vi "validate classes.vi"(6 "Child":refnum<class>, 8 "error in":errorcluster, 11 "Parent":refnum<class>) -> (0 "error out":errorcluster, 1 "class name":string, 3 "unique parent name":string)   [LabVIEW 2020, in "Publisher Subscriber.lvlib"]
uses:
  Publisher Subscriber.lvlib
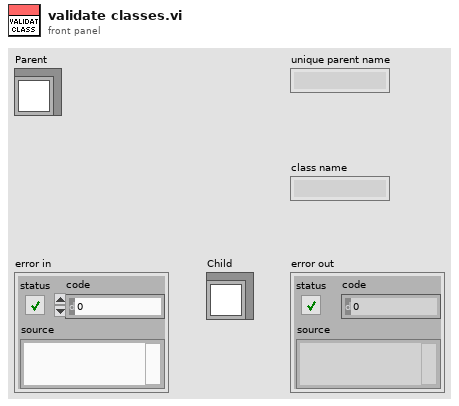
[diagram p1: front panel]
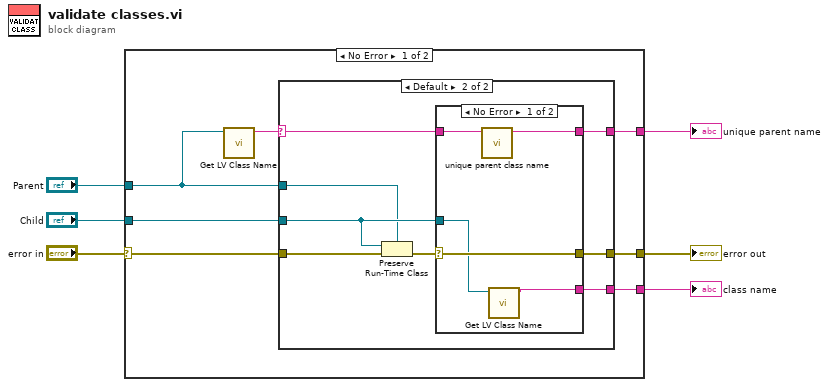
[diagram p0: block diagram]
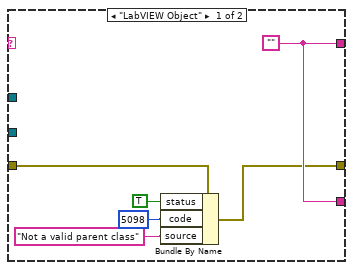
[diagram p2: hidden frame]
diagram:
  n1 = case shown="No Error" "error in" {
    selector: "error in" -> [w7 w34]
    tunnel: [w12 _] -> w6
    tunnel: "Child" -> [w11 _]
    tunnel: [w10 w34] -> w4
    tunnel: "Parent" -> [w9 _]
    tunnel: [w8 _] -> w2
    frame No Error {
      n2 = call <vilib>:"Get LV Class Name.vi"("object"=w9) -> ("class name"=w13:string)  [unwired: 9 in, 1 out]
      n3 = case shown="Default" w13 {
        selector: w13 -> [_ w27]
        tunnel: [w19 w24] -> w12
        tunnel: w11 -> [_ w23]
        tunnel: [w18 w22] -> w10
        tunnel: w9 -> [_ w20]
        tunnel: [w19 w26] -> w8
        tunnel: w7 -> [w17 w25]
        frame "LabVIEW Object" {
          w19 = ""
          n4 = Bundle By Name(cluster=w17, "status"=TRUE, "code"=5098, "source"="Not a valid parent class") -> (w18:errorcluster)
        }
        frame Default {
          n5 = Preserve Run-Time Class(object in=w23, error in=w25, 2:w20) -> (error out=w21:errorcluster)  [unwired: 1 out]
          n6 = case shown="No Error" w21 {
            selector: w21 -> [w29 w33]
            tunnel: w27 -> [w32 _]
            tunnel: [w31 _] -> w26
            tunnel: [w30 _] -> w24
            tunnel: w23 -> [w28 _]
            tunnel: [w29 w33] -> w22
            frame No Error {
              n7 = call "unique parent class name.vi"("class name"=w32) -> ("String"=w30:string)  [unwired: 10 in]
              n8 = call <vilib>:"Get LV Class Name.vi"("object"=w28) -> ("class name"=w31:string)  [unwired: 9 in, 1 out]
            }
            frame Error {
            }
          }
        }
      }
    }
    frame Error {
    }
  }
  "error out" <- w4
  "unique parent name" <- w6
  "class name" <- w2
